vi "Do.vi"(8 "error in (no error)":errorcluster, 10 "Actor in":refnum<class "Actor.lvclass">, 11 "DUTMotor Actor Msg":refnum<class "DUTMotor Actor Msg.lvclass">) -> (0 "error out":errorcluster, 2 "Actor out":refnum<class "Actor.lvclass">)   [LabVIEW 2024, in "DUTMotor Actor.lvlib" / "DUTMotor Actor Msg.lvclass"]
doc: "<p>(<strong>Filename</strong>: <span class=\"dnl\">Actor Framework.lvlib:Message.lvclass:Do.vi</span>)</p>\n<p>Defines what a message does when it is received by an actor. Generally, a message instructs an actor to invoke one of its methods. By default, this method does nothing. A child class must override it to define behavior.</p>"
uses:
  DUTMotor Actor Msg.lvclass
  <vilib>/ActorFramework/Actor/Actor.lvclass
  DUTMotor/DUTMotor.lvclass
  C:/Program Files (x86)/National Instruments/LabVIEW 2024/vi.lib/ActorFramework/Actor/Actor.lvclass
  DUTMotor Actor Msg.lvclass/DUTMotor Actor Msg.ctl
  <vilib>/ActorFramework/Message/Message.lvclass
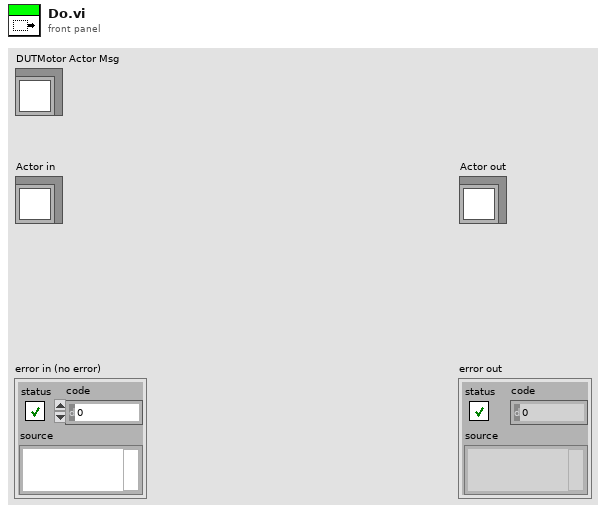
[diagram p1: front panel]
types:
  T1 = typedef "DUTMotorMsgFunc.ctl" = enum16{"StartQuery", "StopQuery", "ConfigMeasData"}
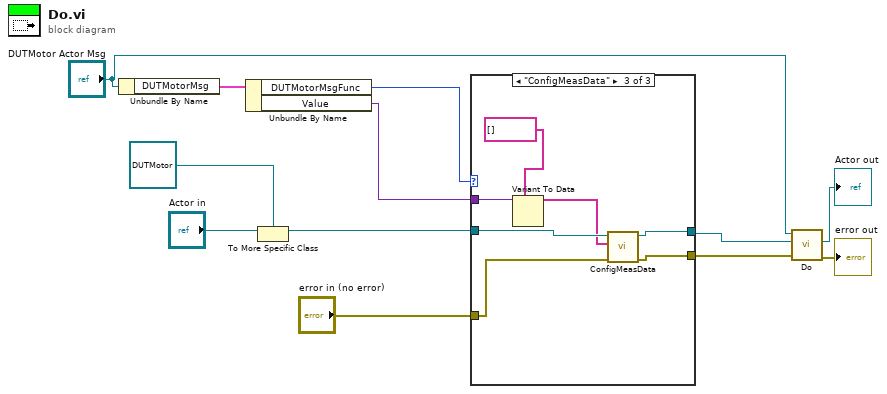
[diagram p0: block diagram]
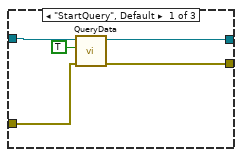
[diagram p2: hidden frame]
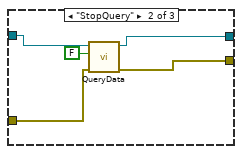
[diagram p3: hidden frame]
diagram:
  n1 = Unbundle By Name("DUTMotor Actor Msg") -> ("DUTMotorMsg"=w10:cluster{"DUTMotorMsgFunc":T1, "Value":variant})
  n2 = Unbundle By Name(w10) -> ("DUTMotorMsgFunc"=w9:T1, "Value"=w1:variant)
  n3 = To More Specific Class(target class=refnum<class "DUTMotor.lvclass"> refnum ("DUTMotor Actor.lvlib:DUTMotor.lvclass"), reference="Actor in") -> (specific class reference=w6:refnum<class "DUTMotor.lvclass">)  [unwired: 1 in, 1 out]
  n4 = case shown="\"ConfigMeasData\"" w9 {
    tunnel: w6 -> [w17 w21 w29]
    tunnel: "error in (no error)" -> [w16 w20 w27]
    tunnel: [w15 w18 w26] -> w4
    tunnel: [w14 w19 w28] -> w3
    tunnel: w1 -> [_ _ w25]
    frame "StartQuery", Default {
      n5 = call "QueryData.vi"("error in (no error)"=w16, "Query?"=TRUE, "DUTMotor in"=w17) -> ("error out"=w15:errorcluster, "DUTMotor out"=w14:refnum<class "DUTMotor.lvclass">)  [unwired: 7 in]
    }
    frame "StopQuery" {
      n6 = call "QueryData.vi"("error in (no error)"=w20, "Query?"=FALSE, "DUTMotor in"=w21) -> ("error out"=w18:errorcluster, "DUTMotor out"=w19:refnum<class "DUTMotor.lvclass">)  [unwired: 7 in]
    }
    frame "ConfigMeasData" {
      n7 = Variant To Data(type=string[] [], Variant=w25) -> (data=w23:string[])  [unwired: 1 in, 1 out]
      n8 = call "ConfigMeasData.vi"("error in (no error)"=w27, "ColumnName"=w23, "DUTMotor in"=w29) -> ("error out"=w26:errorcluster, "DUTMotor out"=w28:refnum<class "DUTMotor.lvclass">)  [unwired: 7 in]
    }
  }
  n9 = call-parent "Do.vi"("error in (no error)"=w4, "Actor in"=w3, "Message"="DUTMotor Actor Msg") -> ("error out"=→"error out":errorcluster, "Actor out"=→"Actor out":refnum<class "Actor.lvclass">)  [unwired: 7 in]
